vi "Average_Array.vi"(2 "Array":dbl[][](array[numeric]), 3 "Ncolumns":i32, 4 "Nrows":i32) -> (0 "Max-Min":dbl[](array[numeric]), 1 "Average":dbl[](array[numeric]))   [LabVIEW 2019]
doc: "Compute the average of the data stored in the columns of an array\n\nNrows = No. of sweeps\nNcolumns = No. data points in each sweep\n\nR. Sheehan 5 - 11 - 2016"
uses:
  <vilib>/Analysis/baseanly.llb/Mean (DBL).vi
  <vilib>/Analysis/NI_AALBase.lvlib
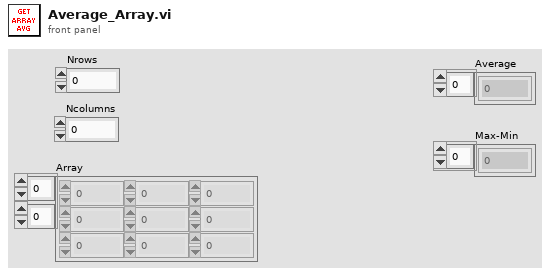
[diagram p1: front panel]
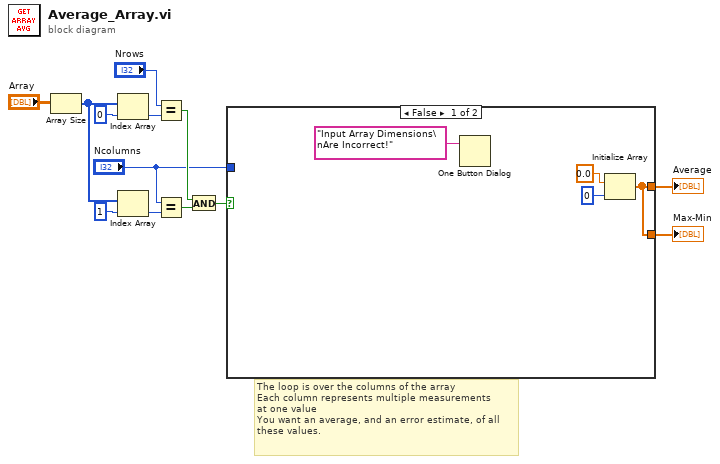
[diagram p0: block diagram]
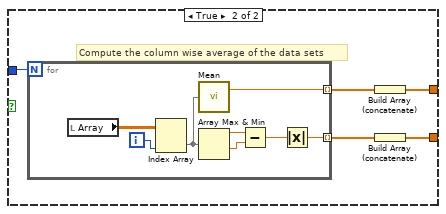
[diagram p2: hidden frame]
diagram:
  # "The loop is over the columns of the array\nEach column represents multiple measurements\nat one value\nYou want an average, and an error estimate, of all\nthese values."
  n1 = Array Size(array="Array") -> (size(s)=w11:i32[])
  n2 = Index Array(array=w11, index=0) -> (element=w10:i32)
  n3 = Index Array(array=w11, index=1) -> (element=w9:i32)
  n4 = Equal?(x="Nrows", y=w10) -> (x = y?=w8:bool)
  n5 = Equal?(x="Ncolumns", y=w9) -> (x = y?=w7:bool)
  n6 = And(x=w8, y=w7) -> (x .and. y?=w6:bool)
  n7 = case shown="False" w6 {
    tunnel: "Ncolumns" -> [_ w20]
    tunnel: [w14 w19] -> w2
    tunnel: [w14 w18] -> w1
    frame False {
      n8 = One Button Dialog(message="Input Array Dimensions\nAre Incorrect!") -> ()  [unwired: 1 in, 1 out]
      n9 = Initialize Array(0.0 ("element"), 0 ("dimension size")) -> (w14:dbl[])
    }
    frame True {
      # "Compute the column wise average of the data sets"
      n10 = for {
        N: w20 -> [_]
        tunnel: [w28] -> w21 mode=indexing
        tunnel: [w23] -> w22 mode=indexing
        i -> [w29]
        n11 = local read "Array"() -> (w30:dbl[][])
        n12 = Index Array(array=w30, index (col)=w29) -> (element=w27:dbl[])  [unwired: 1 in]
        n13 = call-poly <vilib>:"Mean.vi"("X"=w27) -> ("mean"=w28:dbl)  [unwired: 1 out]
        n14 = Array Max & Min(array=w27) -> (max value=w25:dbl, min value=w26:dbl)  [unwired: 2 out]
        n15 = Subtract(x=w25, y=w26) -> (x-y=w24:dbl)
        n16 = Absolute Value(x=w24) -> (abs(x)=w23:dbl)
      }
      n17 = Build Array (concatenate)(w21) -> (w19:dbl[])
      n18 = Build Array (concatenate)(w22) -> (w18:dbl[])
    }
  }
  "Average" <- w2
  "Max-Min" <- w1
